vi "Get Value Node.vi"(7 "Data Type":T1=enum."String", 8 "error in":errorcluster, 9 "Key":string, 10 "Section":string, 11 "Root Node":variant) -> (0 "error out":errorcluster, 2 "Value Node out":variant)   [LabVIEW 2022 SP3, in "hse-config.lvlib" / "config-base.lvclass"]
doc: "Returns a value node (a Variant) of the given Section an Key.\n\n____\nHAMPEL SOFTWARE ENGINEERING v3.8.0 (2023-12-18 14:41)"
uses:
  config-base.lvclass
  <vilib>/Utility/Data Type/Type Definitions/Data Type.ctl
  <vilib>/Utility/Data Type/NI_Data Type.lvlib
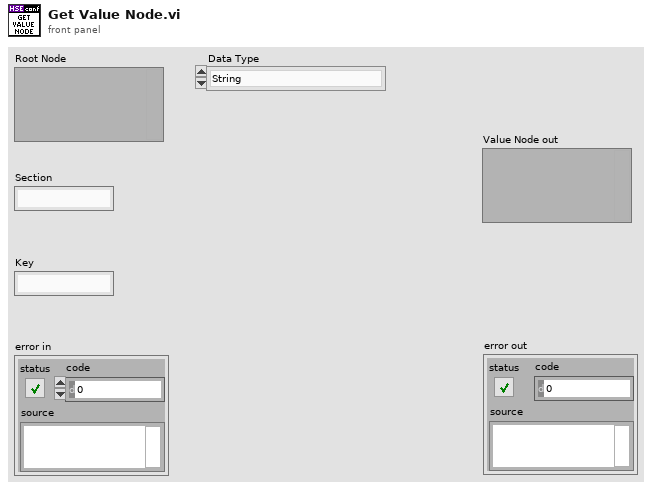
[diagram p1: front panel]
types:
  T1 = typedef "NI_Data Type.lvlib/Data Type.ctl" = enum8{"Invalid Type", "Void", "I8", "I16", "I32", "I64", "U8", "U16", "U32", "U64", "Single Float", "Double Float", "Extended Float", "Single Complex", "Double Complex", "Extended Complex", "Enum U8", "Enum U16", "Enum U32", "Enum U64", "Single Float With Unit", "Double Float With Unit", "Extended Float With Unit", "Single Complex with Unit", "Double Complex with Unit", "Extended Complex with Unit", "Boolean", "String", "Path", "Picture", "Tag", "Array", "Cluster", "Variant", "LV Variant", "Waveform", "Timestamp", "Digital Waveform", "Digital Data", "ExpressData", "Refnum", "External Data", "VI", "Poly VI", "LabVIEW Class Instance", "Fixed Point", "Set Collection", "Map Collection"}
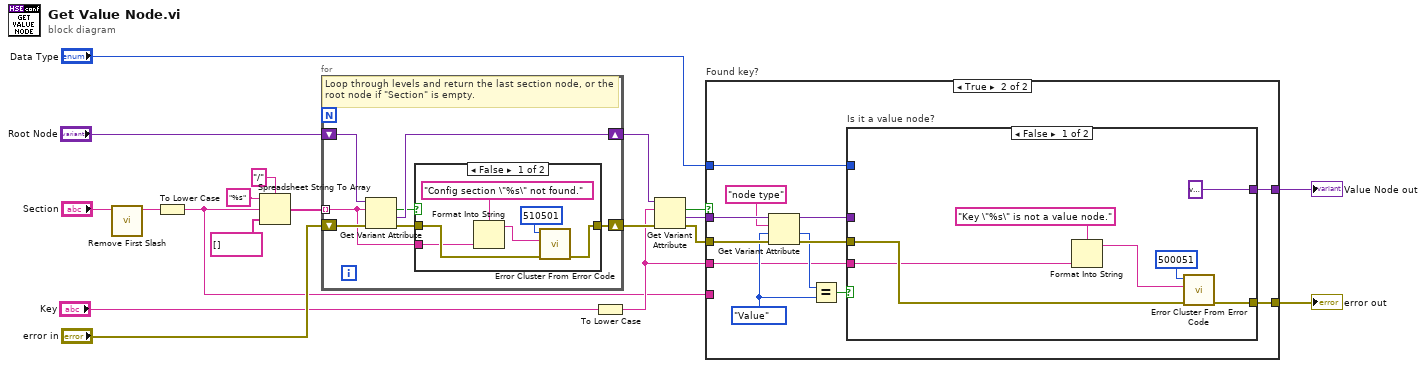
[diagram p0: block diagram]
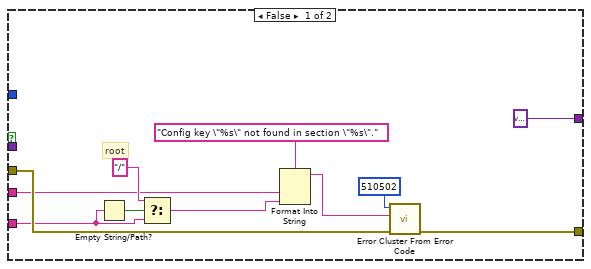
[diagram p2: hidden frame]
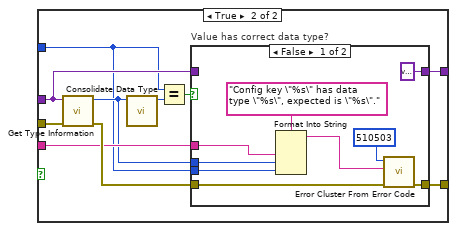
[diagram p3: hidden frame]
diagram:
  n1 = call "Remove First Slash.vi"("Section"="Section") -> ("result string"=w4:string)  [unwired: 10 in]
  n2 = To Lower Case(string=w4) -> (all lower case string=w1:string)
  n3 = Spreadsheet String To Array(delimiter (Tab)="/" ("Split Pattern"), format string="%s", spreadsheet string=w1, array type (2D Dbl)=string[] []) -> (array=w12:string[])
  n4 = for {
    shift-right: [w21] -> w16
    shift-left: "error in" -> [w25]
    tunnel: w12 -> [w20] mode=indexing
    shift-right: [w24] -> w11
    shift-left: "Root Node" -> [w26]
    # "Loop through levels and return the last section node, or the root node if \"Section\" is empty."
    n5 = Get Variant Attribute(Variant=w26, name=w20, error in=w25) -> (found=w22:bool, value=w24:variant, error out=w23:errorcluster)  [unwired: 1 in, 1 out]
    n6 = case shown="False" w22 {
      tunnel: w23 -> [w32 w33]
      tunnel: [w31 w33] -> w21
      tunnel: w20 -> [w27 _]
      frame False {
        n7 = Format Into String(format string="Config section \"%s\" not found.", w27) -> (resulting string=w28:string)  [unwired: 2 in, 1 out]
        n8 = call <vilib>:"Error Cluster From Error Code.vi"("error in (no error)"=w32, "error message (\"\")"=w28, "error code (0)"=510501) -> ("error out"=w31:errorcluster)  [unwired: 6 in]
      }
      frame True {
      }
    }
  }
  n9 = To Lower Case(string="Key") -> (all lower case string=w2:string)
  n10 = Get Variant Attribute(Variant=w11, name=w2, error in=w16) -> (found=w10:bool, value=w9:variant, error out=w7:errorcluster)  [unwired: 1 in, 1 out]
  n11 = case "Found key?" shown="True" w10 {
    tunnel: w7 -> [w41 w54]
    tunnel: w9 -> [_ w55]
    tunnel: w2 -> [w35 w47]
    tunnel: "Data Type" -> [_ w48]
    tunnel: [variant w46] -> w5
    tunnel: [w40 w45] -> w17
    tunnel: w1 -> [w36 _]
    frame False {
      # "root"
      n12 = Empty String/Path?(string/path=w36) -> (empty?=w38:bool)
      n13 = Select(t="/", s=w38, f=w36) -> (s? t:f=w34:string)
      n14 = Format Into String(format string="Config key \"%s\" not found in section \"%s\".", w35, w34) -> (resulting string=w42:string)  [unwired: 2 in, 1 out]
      n15 = call <vilib>:"Error Cluster From Error Code.vi"("error in (no error)"=w41, "error message (\"\")"=w42, "error code (0)"=510502) -> ("error out"=w40:errorcluster)  [unwired: 6 in]
    }
    frame True {
      w51 = enum8{"Root", "Section", "Value"}."Value" ("Node Type")
      n16 = Get Variant Attribute(Variant=w55, name="node type", default value (empty Variant)=w51, error in=w54) -> (duplicate Variant=w50:variant, value=w52:enum8{"Root", "Section", "Value"}, error out=w56:errorcluster)  [unwired: 1 out]
      n17 = Equal?(x=w52, y=w51) -> (x = y?=w49:bool)
      n18 = case "Is it a value node?" shown="False" w49 {
        tunnel: w56 -> [w61 w72]
        tunnel: w50 -> [_ w70]
        tunnel: w48 -> [_ w64]
        tunnel: w47 -> [w57 w69]
        tunnel: [variant w68] -> w46
        tunnel: [w62 w67] -> w45
        frame False {
          n19 = Format Into String(format string="Key \"%s\" is not a value node.", w57) -> (resulting string=w60:string)  [unwired: 2 in, 1 out]
          n20 = call <vilib>:"Error Cluster From Error Code.vi"("error in (no error)"=w61, "error message (\"\")"=w60, "error code (0)"=500051) -> ("error out"=w62:errorcluster)  [unwired: 6 in]
        }
        frame True {
          n21 = call <vilib>:"Get Type Information.vi"("error in (no error)"=w72, "variant"=w70) -> ("error out"=w73:errorcluster, "type"=w66:T1)  [unwired: 5 in, 3 out]
          n22 = call "Consolidate Data Type.vi"("Type in"=w66) -> ("Type out"=w65:T1)  [unwired: 10 in]
          n23 = Equal?(x=w64, y=w65) -> (x = y?=w71:bool)
          n24 = case "Value has correct data type?" shown="False" w71 {
            tunnel: w73 -> [w82 w83]
            tunnel: w70 -> [_ w84]
            tunnel: [variant w84] -> w68
            tunnel: [w78 w83] -> w67
            tunnel: w64 -> [w77 _]
            tunnel: w66 -> [w76 _]
            tunnel: w69 -> [w75 _]
            frame False {
              n25 = Format Into String(format string="Config key \"%s\" has data type \"%s\", expected is \"%s\".", w75, w76, w77) -> (resulting string=w80:string)  [unwired: 2 in, 1 out]
              n26 = call <vilib>:"Error Cluster From Error Code.vi"("error in (no error)"=w82, "error message (\"\")"=w80, "error code (0)"=510503) -> ("error out"=w78:errorcluster)  [unwired: 6 in]
            }
            frame True {
            }
          }
        }
      }
    }
  }
  "Value Node out" <- w5
  "error out" <- w17
